vi "RS_generator_modulation.vi"(1 "Generator Output":bool=TRUE, 2 "Modulation Depth (%)":sgl=100.0 min=0 max=100 step=0.01, 3 "Modulation Frequency (Hz)":u64=100000, 4 "address":string="192.168.0.7") -> ()   [LabVIEW 2013]
panel:
  out "resulting string":string
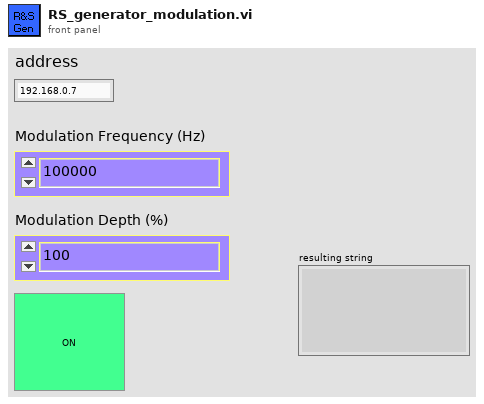
[diagram p1: front panel]
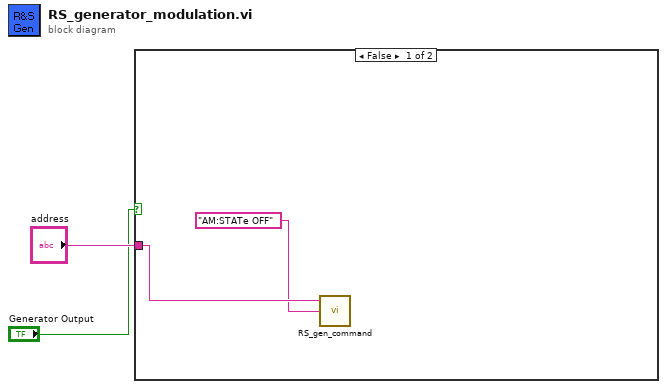
[diagram p0: block diagram]
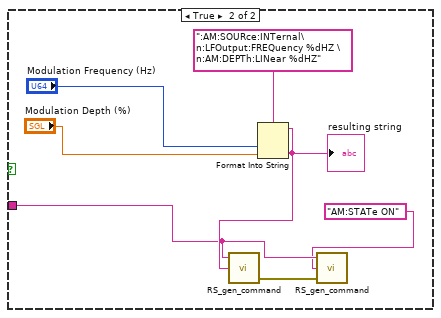
[diagram p2: hidden frame]
diagram:
  n1 = case shown="False" "Generator Output" {
    tunnel: "address" -> [w4 w6]
    frame False {
      n2 = call "RS_gen_command.vi"("Comand"="AM:STATe OFF" ("string"), "address"=w4) -> ()  [unwired: 3 in, 1 out]
    }
    frame True {
      n3 = Format Into String(format string=":AM:SOURce:INTernal\n:LFOutput:FREQuency %dHZ \n:AM:DEPTh:LINear %dHZ" ("string"), "Modulation Frequency (Hz)", "Modulation Depth (%)") -> (resulting string=w8:string)  [unwired: 2 in, 1 out]
      "resulting string" <- w8
      n4 = call "RS_gen_command.vi"("Comand"=w8, "address"=w6) -> ("error out"=w7:errorcluster)  [unwired: 3 in]
      n5 = call "RS_gen_command.vi"("error in (no error)"=w7, "Comand"="AM:STATe ON" ("string"), "address"=w6) -> ()  [unwired: 2 in, 1 out]
    }
  }
